vi "Vision Target Global.vi"() -> ()   [LabVIEW 2016, in "Vision Drive.lvlib"]
uses:
  Vision Drive.lvlib
  Target to Robot.ctl
panel:
  in  "Target":T1
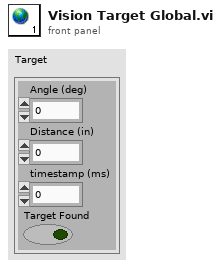
[diagram p1: front panel]
types:
  T1 = typedef "Vision Drive.lvlib/Target to Robot.ctl" = cluster{"Angle (deg)":dbl, "Distance (in)":dbl, "timestamp (ms)":u32, "Target Found":bool}
diagram:
